vi "If there is no reading stop acc.vi"(2 "Last Pedals Update":u32, 9 "\"Pedals\" Status in":T1 {"Acceleration pedal" scale=0.0..100.0 scale format="%#_6f%%"; "Break pedal" scale=0.0..100.0 scale format="%#_6f%%"}, 10 "Update Motors Notifier":refnum<notifier>) -> (1 "\"Pedals\" Status out":T1 {"Acceleration pedal" scale=0.0..100.0 scale format="%#_6f%%"; "Break pedal" scale=0.0..100.0 scale format="%#_6f%%"})   [LabVIEW 2016]
uses:
  RT/Pedals Status.ctl
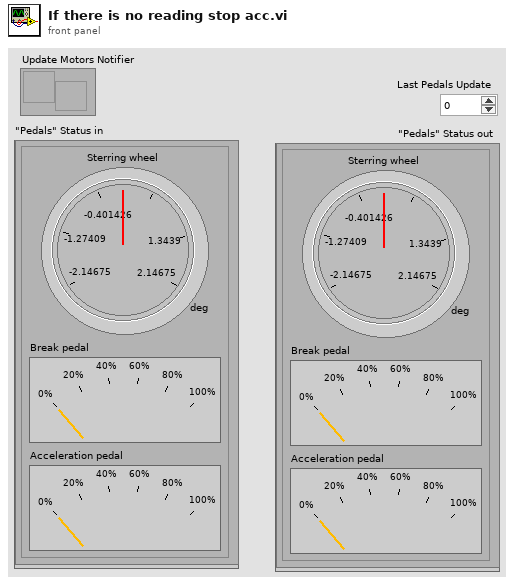
[diagram p1: front panel]
types:
  T1 = typedef "Pedals Status.ctl" = cluster{"Acceleration pedal":dbl, "Break pedal":dbl, "Sterring wheel":dbl[unit]}
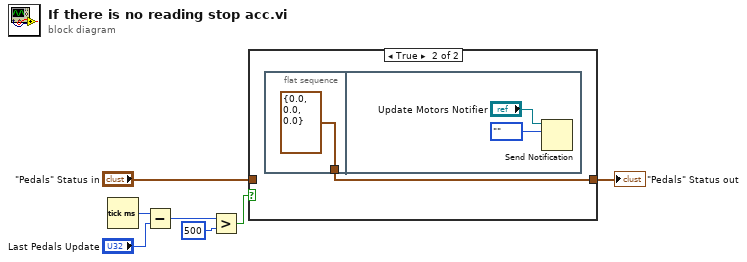
[diagram p0: block diagram]
diagram:
  n1 = Tick Count (ms)() -> (millisecond timer value=w7:u32)
  n2 = Subtract(x=w7, y="Last Pedals Update") -> (x-y=w6:u32)
  n3 = Greater?(x=w6, y=u32 500) -> (0:w4:bool)
  n4 = case shown="True" w4 {
    tunnel: [w8 w9] -> w2
    tunnel: "\"Pedals\" Status in" -> [w8 _]
    frame False {
    }
    frame True {
      n5 = flat-sequence {
        tunnel: [T1 {"Acceleration pedal"=0.0, "Break pedal"=0.0, "Sterring wheel"=0.0} ("\"Pedals\" Status")] -> w9
        frame #0 {
        }
        frame #1 {
          n6 = Send Notification(notification=enum16{""}."", notifier="Update Motors Notifier") -> ()  [unwired: 1 in, 2 out]
        }
      }
    }
  }
  "\"Pedals\" Status out" <- w2
